vi "MidbrainBehaviorEngine.vi"(11 "ForebrainCom":T2) -> (0 "BehaviorInhibit":T1, 3 "VelCom":dbl)   [LabVIEW 2012]
doc: "This sub VI takes the commanded mission velocity and robot behavior from the Forebrain and activates the appropriate Midbrain subbehaviors to cary it out."
panel:
  # "This subVI takes the current desired robot\nvelocity andoverall  behavior from the Forebrain\nand activates the appropriate Midbrain sub-behaviors\nto carry it out"
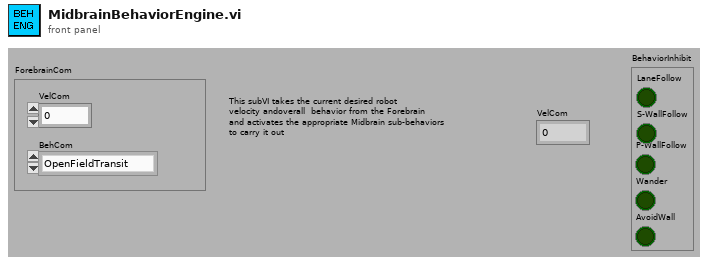
[diagram p1: front panel]
types:
  T1 = cluster{"AvoidWall":bool, "Wander":bool, "P-WallFollow":bool, "LaneFollow":bool, "S-WallFollow":bool}
  T2 = cluster{"VelCom":dbl, "BehCom":enum16{"OpenFieldTransit", "P-WallFollow", "S-WallFollow", "LaneFollow", "ManualMode"}}
  T3 = enum16{"OpenFieldTransit", "P-WallFollow", "S-WallFollow", "LaneFollow", "ManualMode"}
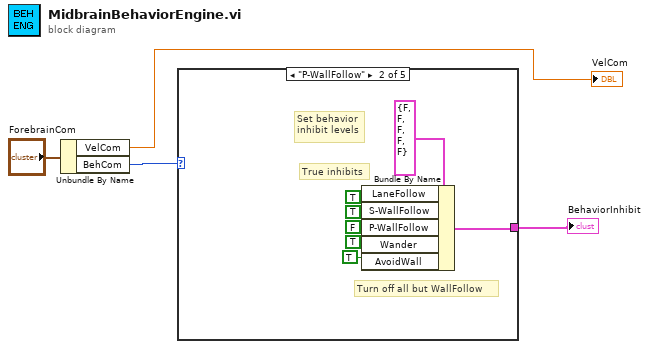
[diagram p0: block diagram]
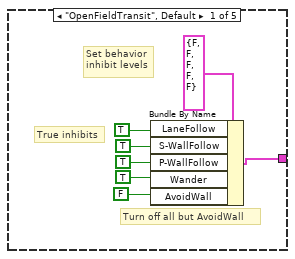
[diagram p2: hidden frame]
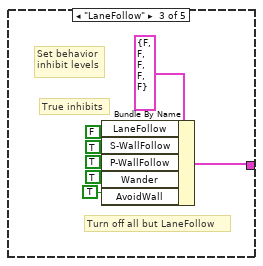
[diagram p3: hidden frame]
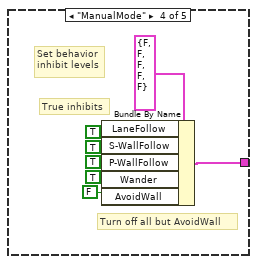
[diagram p4: hidden frame]
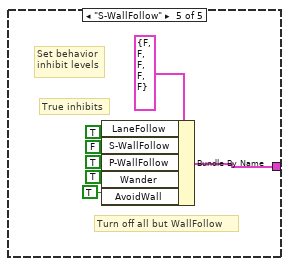
[diagram p5: hidden frame]
diagram:
  n1 = Unbundle By Name("ForebrainCom") -> ("VelCom"=→"VelCom":dbl, "BehCom"=w2:T3)
  n2 = case shown="\"P-WallFollow\"" w2 {
    tunnel: [w6 w12 w19 w26 w33] -> w1
    frame "OpenFieldTransit", Default {
      # "True inhibits"
      # "Set behavior\ninhibit levels"
      # "Turn off all but AvoidWall"
      n3 = Bundle By Name(cluster=T1 {"AvoidWall"=FALSE, "Wander"=FALSE, "P-WallFollow"=FALSE, "LaneFollow"=FALSE, "S-WallFollow"=FALSE} ("BehaviorInhibit"), "LaneFollow"=TRUE, "S-WallFollow"=TRUE ("WallFollow"), "P-WallFollow"=TRUE ("Wander"), "Wander"=TRUE ("AvoidWall"), "AvoidWall"=FALSE) -> (w6:T1)
    }
    frame "P-WallFollow" {
      # "True inhibits"
      # "Set behavior\ninhibit levels"
      # "Turn off all but WallFollow"
      n4 = Bundle By Name(cluster=T1 {"AvoidWall"=FALSE, "Wander"=FALSE, "P-WallFollow"=FALSE, "LaneFollow"=FALSE, "S-WallFollow"=FALSE} ("BehaviorInhibit"), "LaneFollow"=TRUE, "S-WallFollow"=TRUE ("WallFollow"), "P-WallFollow"=FALSE ("Wander"), "Wander"=TRUE ("AvoidWall"), "AvoidWall"=TRUE) -> (w12:T1)
    }
    frame "LaneFollow" {
      # "True inhibits"
      # "Set behavior\ninhibit levels"
      # "Turn off all but LaneFollow"
      n5 = Bundle By Name(cluster=T1 {"AvoidWall"=FALSE, "Wander"=FALSE, "P-WallFollow"=FALSE, "LaneFollow"=FALSE, "S-WallFollow"=FALSE} ("BehaviorInhibit"), "LaneFollow"=FALSE, "S-WallFollow"=TRUE ("WallFollow"), "P-WallFollow"=TRUE ("Wander"), "Wander"=TRUE ("AvoidWall"), "AvoidWall"=TRUE) -> (w19:T1)
    }
    frame "ManualMode" {
      # "True inhibits"
      # "Set behavior\ninhibit levels"
      # "Turn off all but AvoidWall"
      n6 = Bundle By Name(cluster=T1 {"AvoidWall"=FALSE, "Wander"=FALSE, "P-WallFollow"=FALSE, "LaneFollow"=FALSE, "S-WallFollow"=FALSE} ("BehaviorInhibit"), "LaneFollow"=TRUE, "S-WallFollow"=TRUE ("WallFollow"), "P-WallFollow"=TRUE ("Wander"), "Wander"=TRUE ("AvoidWall"), "AvoidWall"=FALSE) -> (w26:T1)
    }
    frame "S-WallFollow" {
      # "True inhibits"
      # "Set behavior\ninhibit levels"
      # "Turn off all but WallFollow"
      n7 = Bundle By Name(cluster=T1 {"AvoidWall"=FALSE, "Wander"=FALSE, "P-WallFollow"=FALSE, "LaneFollow"=FALSE, "S-WallFollow"=FALSE} ("BehaviorInhibit"), "LaneFollow"=TRUE, "S-WallFollow"=FALSE ("WallFollow"), "P-WallFollow"=TRUE ("Wander"), "Wander"=TRUE ("AvoidWall"), "AvoidWall"=TRUE) -> (w33:T1)
    }
  }
  "BehaviorInhibit" <- w1
